vi "Write VI Refnum-Main.vi"(8 "error in (no error)":errorcluster, 10 "VI Refnum-Main":refnum<vi>, 11 "Result Info in":refnum<class "Result Info.lvclass">) -> (0 "error out":errorcluster, 3 "Result Info out":refnum<class "Result Info.lvclass">)   [LabVIEW 2023, in "Data Analysis.lvlib" / "Result Info.lvlib" / "Result Info.lvclass"]
uses:
  Result Info.lvclass
  Result Info.lvclass/Result Info.ctl
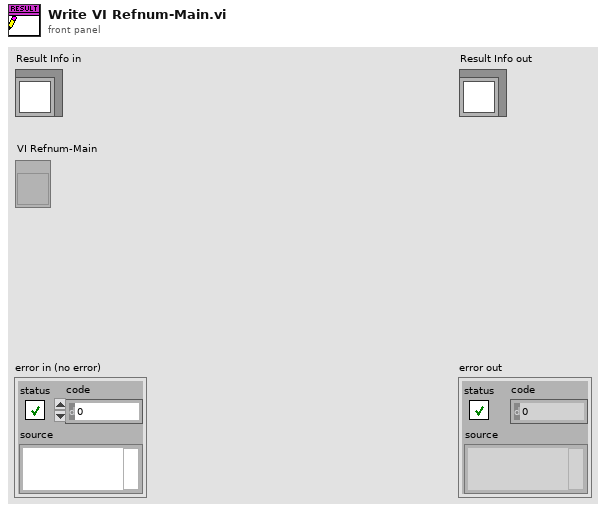
[diagram p1: front panel]
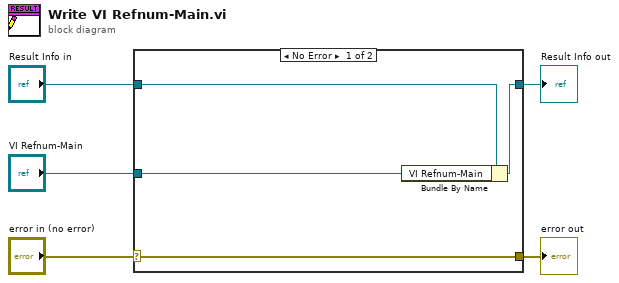
[diagram p0: block diagram]
diagram:
  n1 = case shown="No Error" "error in (no error)" {
    selector: "error in (no error)" -> [w9 w10]
    tunnel: [w9 w10] -> w4
    tunnel: [w7 w11] -> w2
    tunnel: "Result Info in" -> [w8 w11]
    tunnel: "VI Refnum-Main" -> [w6 _]
    frame No Error {
      n2 = Bundle By Name(cluster=w8, "VI Refnum-Main"=w6) -> (w7:refnum<class "Result Info.lvclass">)
    }
    frame Error {
    }
  }
  "error out" <- w4
  "Result Info out" <- w2
